vi "Access DB Path.vi"(10 "ping":bool, 11 "database":string="database1.mdb") -> (2 "Connection information":string, 3 "Path out":string)   [LabVIEW 2016, in "Access Lib.lvlib"]
uses:
  Access Lib.lvlib
  <vilib>/Utility/sysdir.llb/System Directory Type.ctl
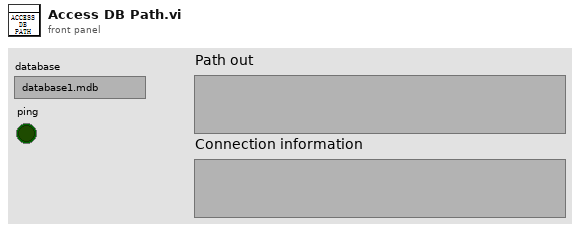
[diagram p1: front panel]
types:
  T1 = typedef "System Directory Type.ctl" = i32
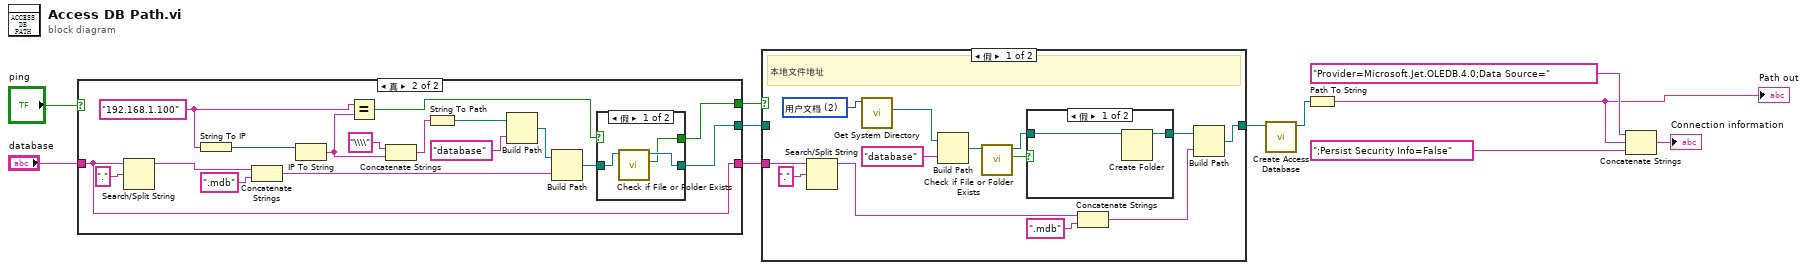
[diagram p0: block diagram]
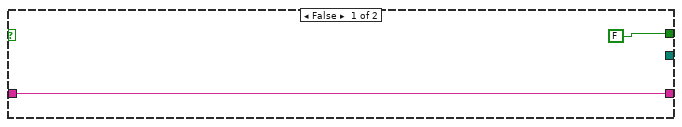
[diagram p4: hidden frame]
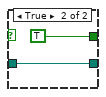
[diagram p5: hidden frame]
diagram:
  n1 = case shown="真" "ping" {
    tunnel: [_ w21] -> w7
    tunnel: [FALSE ("file or folder exists?") w20] -> w8
    tunnel: [w12 w14] -> w9
    tunnel: "database" -> [w12 w14]
    frame False {
    }
    frame True {
      w19 = "192.168.1.100" ("名称")
      n2 = Search/Split String(string=w14, search string/char (-)="." ("搜索字符串/字符(-)")) -> (substring before match=w18:string)  [unwired: 1 in, 2 out]
      n3 = String To IP(1:w19) -> (0:w30:u32)
      n4 = Concatenate Strings(w18, ".mdb" ("字符串")) -> (w15:string)
      n5 = IP To String(2:w30) -> (0:w24:string)  [unwired: 1 in]
      n6 = Equal?(x=w19, y=w24) -> (x = y?=w23:bool)
      n7 = Concatenate Strings("\\\\" ("字符串"), w24) -> (w27:string)
      n8 = String To Path(string=w27) -> (path=w29:path)
      n9 = Build Path(base path=w29, name or relative path="database" ("名称或相对路径")) -> (appended path=w25:path)
      n10 = Build Path(base path=w25, name or relative path=w15) -> (appended path=w22:path)
      n11 = case shown="假" w23 {
        tunnel: w22 -> [w33 w34]
        tunnel: [w32 w34] -> w21
        tunnel: [w31 TRUE] -> w20
        frame False {
          n12 = call <vilib>:"Check if File or Folder Exists.vi"("path"=w33) -> ("file or folder exists?"=w31:bool, "dup path"=w32:path)  [unwired: 8 in, 1 out]
        }
        frame True {
        }
      }
    }
  }
  n13 = case shown="假" w8 {
    tunnel: w9 -> [w38 _]
    tunnel: [w36 w52] -> w11
    tunnel: w7 -> [_ w52]
    frame False {
      w45 = T1 2 items=["用户目录"=0, "用户桌面"=1, "用户文档"=2, "用户应用程序数据"=3, "用户设置"=4, "用户临时目录"=5, "公共文档"=6, "公共应用程序数据"=7, "公共设置"=8, "公共缓存"=13, "系统核心库"=9, "系统安装库"=10, "应用程序文件"=11, "启动盘根目录"=12] ("system directory type")
      # "本地文件地址"
      n14 = Search/Split String(string=w38, search string/char (-)="." ("搜索字符串/字符(-)")) -> (substring before match=w41:string)  [unwired: 1 in, 2 out]
      n15 = call <vilib>:"Get System Directory.vi"("system directory type"=w45) -> ("system directory"=w44:path)  [unwired: 10 in]
      n16 = Build Path(base path=w44, name or relative path="database" ("名称或相对路径")) -> (appended path=w42:path)
      n17 = call <vilib>:"Check if File or Folder Exists.vi"("path"=w42) -> ("file or folder exists?"=w48:bool, "dup path"=w47:path)  [unwired: 8 in, 1 out]
      n18 = case shown="假" w48 {
        tunnel: w47 -> [w50 w51]
        tunnel: [w49 w51] -> w46
        frame False {
          n19 = Create Folder(path (use dialog)=w50) -> (created path=w49:path)  [unwired: 2 in, 2 out]
        }
        frame True {
        }
      }
      n20 = Concatenate Strings(w41, ".mdb" ("字符串")) -> (w37:string)
      n21 = Build Path(base path=w46, name or relative path=w37) -> (appended path=w36:path)
    }
    frame True {
      # "共享文件地址"
    }
  }
  n22 = call "Create Access Database.vi"("路径"=w11) -> ("路径 out"=w1:path)  [unwired: 9 in, 1 out]
  n23 = Path To String(path=w1) -> (string=w3:string)
  "Path out" <- w3
  n24 = Concatenate Strings("Provider=Microsoft.Jet.OLEDB.4.0;Data Source=" ("condition"), w3, ";Persist Security Info=False" ("condition")) -> (→"Connection information":string)
